vi "general scan information.vi"(8 "Error In":errorcluster, 10 "General information in":T2={"Operator"="", "Setup"=enum."fiber-coupled", "Sample"="", "Source name"="", "Source current [mA]"=""}, 11 "mode (R)":T1=enum."read") -> (0 "Error out":errorcluster, 2 "general information out":T2={"Operator"="", "Setup"=enum."fiber-coupled", "Sample"="", "Source name"="", "Source current [mA]"=""})   [LabVIEW 2011]
doc: "Functional Global Variable for the algorithm settings. The used method as well as the max. Iteration steps and the tolerance can be given. In addition, the algorithm can be told to use boundaries (if possible)."
uses:
  controls/general information.ctl
  controls/FGV_Action.ctl
panel:
  # "Input"
  # "Output"
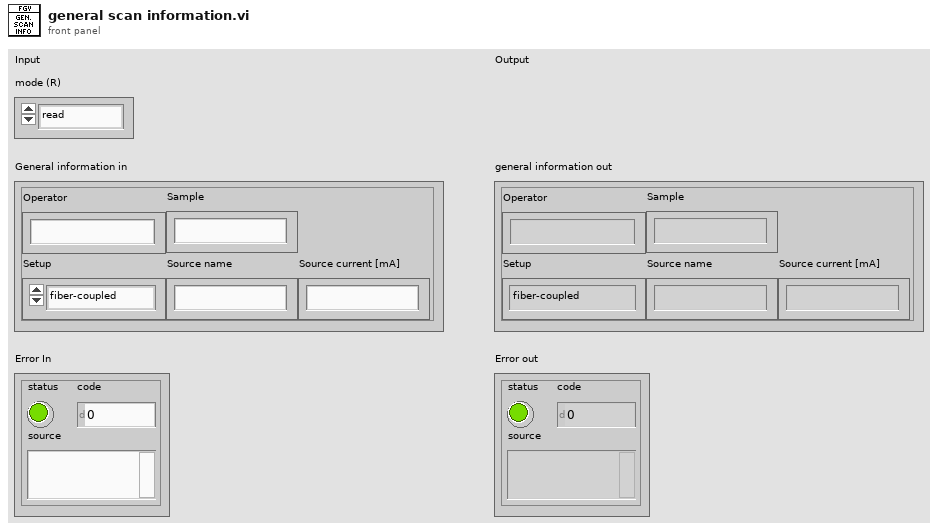
[diagram p1: front panel]
types:
  T1 = typedef "FGV_Action.ctl" = enum16{"set to default", "read", "write"}
  T2 = typedef "general information.ctl" = cluster{"Operator":string, "Setup":enum16{"fiber-coupled (temp. controlled)", "fiber-coupled", "lensed fiber setup (temp. controlled)", "lensed fiber setup"}, "Sample":string, "Source name":string, "Source current [mA]":string}
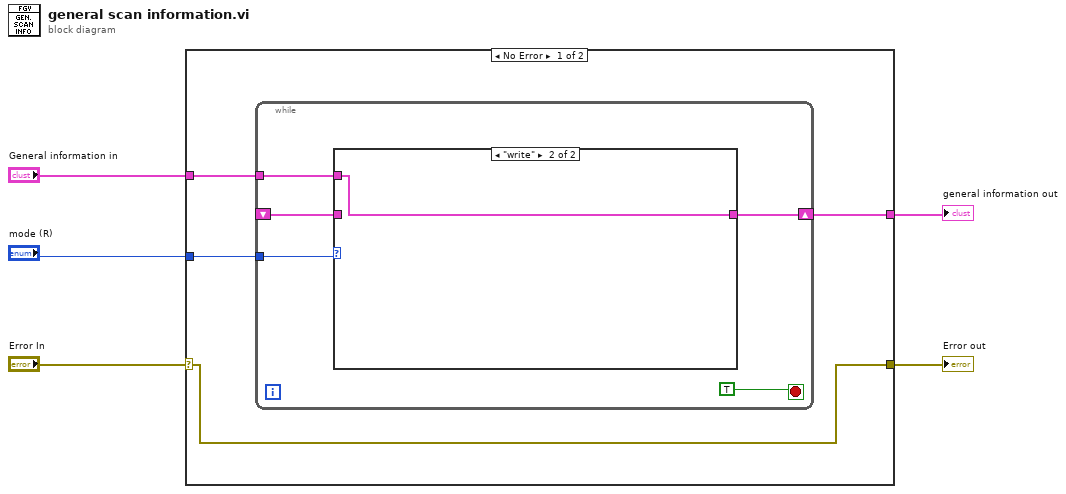
[diagram p0: block diagram]
diagram:
  n1 = case shown="No Error" "Error In" {
    selector: "Error In" -> [w6 w18]
    tunnel: "mode (R)" -> [w9 _]
    tunnel: [w6 w18] -> w4
    tunnel: "General information in" -> [w8 w17]
    tunnel: [w7 w17] -> w2
    frame No Error {
      n2 = while {
        tunnel: w9 -> [w13]
        tunnel: w8 -> [w12]
        shift-right: [w10] -> w7
        shift-left: _ -> [w11]
        stop <- TRUE stop-if-true
        n3 = case shown="\"write\"" w13 {
          tunnel: w12 -> [_ w16]
          tunnel: w11 -> [w15 _]
          tunnel: [w15 w16] -> w10
          frame "read", Default {
          }
          frame "write" {
          }
        }
      }
    }
    frame Error {
    }
  }
  "Error out" <- w4
  "general information out" <- w2
